vi "Get Random Number bn Min and Max.vi"(0 "Min":i32, 5 "Max":i32) -> (4 "Random Value":i32)   [LabVIEW 2014, in "Dragon Tamers.lvlib"]
uses:
  Dragon Tamers.lvlib
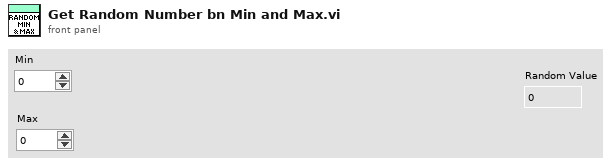
[diagram p1: front panel]
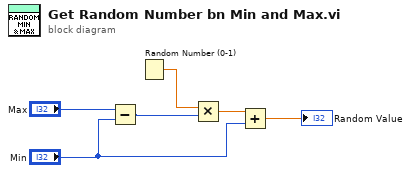
[diagram p0: block diagram]
diagram:
  n1 = Subtract(x="Max", y="Min") -> (x-y=w2:i32)
  n2 = Random Number (0-1)() -> (number: 0 to 1=w5:dbl)
  n3 = Multiply(x=w5, y=w2) -> (x*y=w4:dbl)
  n4 = Add(x=w4, y="Min") -> (x+y=→"Random Value":dbl)
